vi "Config Load Sidestep Globals.vi"(11 "refnum":T1) -> (3 "refnum Out":T1)   [LabVIEW 2012]
uses:
  <vilib>/Utility/config.llb/Config Data RefNum.ctl
  <vilib>/Utility/config.llb/Read Key (Double).vi
  Sidestep Globals.vi
  <vilib>/Utility/config.llb/NI_LVConfig.lvlib
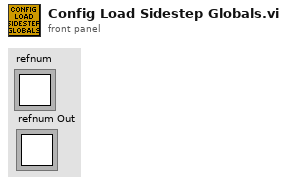
[diagram p1: front panel]
types:
  T1 = typedef "NI_LVConfig.lvlib/Config Data RefNum.ctl" = refnum<k1>
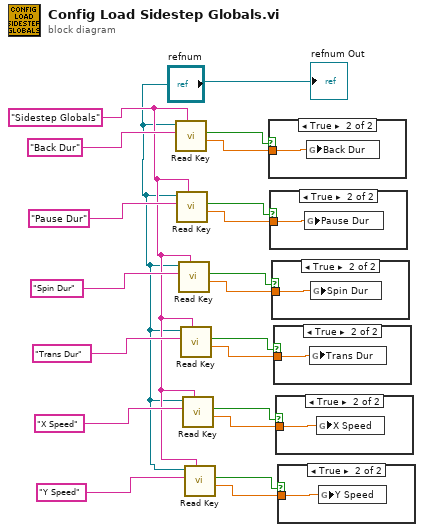
[diagram p0: block diagram]
diagram:
  w2 = "Sidestep Globals"
  n1 = call-poly <vilib>:"Read Key.vi"("section"=w2, "key"="Back Dur", "refnum"="refnum") -> ("value"=w20:dbl, "found?"=w18:bool)  [unwired: 5 in, 2 out]
  n2 = call-poly <vilib>:"Read Key.vi"("section"=w2, "key"="Pause Dur", "refnum"="refnum") -> ("value"=w15:dbl, "found?"=w17:bool)  [unwired: 5 in, 2 out]
  n3 = call-poly <vilib>:"Read Key.vi"("section"=w2, "key"="Spin Dur", "refnum"="refnum") -> ("value"=w14:dbl, "found?"=w12:bool)  [unwired: 5 in, 2 out]
  n4 = call-poly <vilib>:"Read Key.vi"("section"=w2, "key"="Trans Dur", "refnum"="refnum") -> ("value"=w8:dbl, "found?"=w6:bool)  [unwired: 5 in, 2 out]
  n5 = call-poly <vilib>:"Read Key.vi"("section"=w2, "key"="X Speed", "refnum"="refnum") -> ("value"=w9:dbl, "found?"=w11:bool)  [unwired: 5 in, 2 out]
  n6 = call-poly <vilib>:"Read Key.vi"("section"=w2, "key"="Y Speed", "refnum"="refnum") -> ("value"=w5:dbl, "found?"=w3:bool)  [unwired: 5 in, 2 out]
  n7 = case shown="True" w18 {
    tunnel: w20 -> [_ w21]
    frame False {
    }
    frame True {
      n8 = global write "Sidestep Globals.vi" "Back Dur"(w21) -> ()
    }
  }
  n9 = case shown="True" w17 {
    tunnel: w15 -> [_ w22]
    frame False {
    }
    frame True {
      n10 = global write "Sidestep Globals.vi" "Pause Dur"(w22) -> ()
    }
  }
  n11 = case shown="True" w12 {
    tunnel: w14 -> [_ w23]
    frame False {
    }
    frame True {
      n12 = global write "Sidestep Globals.vi" "Spin Dur"(w23) -> ()
    }
  }
  n13 = case shown="True" w6 {
    tunnel: w8 -> [_ w24]
    frame False {
    }
    frame True {
      n14 = global write "Sidestep Globals.vi" "Trans Dur"(w24) -> ()
    }
  }
  n15 = case shown="True" w11 {
    tunnel: w9 -> [_ w25]
    frame False {
    }
    frame True {
      n16 = global write "Sidestep Globals.vi" "X Speed"(w25) -> ()
    }
  }
  n17 = case shown="True" w3 {
    tunnel: w5 -> [_ w26]
    frame False {
    }
    frame True {
      n18 = global write "Sidestep Globals.vi" "Y Speed"(w26) -> ()
    }
  }
  "refnum Out" <- "refnum"
